vi "waypoint save to file.vi"() -> ()   [LabVIEW 2019]
panel:
  out "XY 그래프":cluster{"X":dbl, "Y":dbl}[](graph)
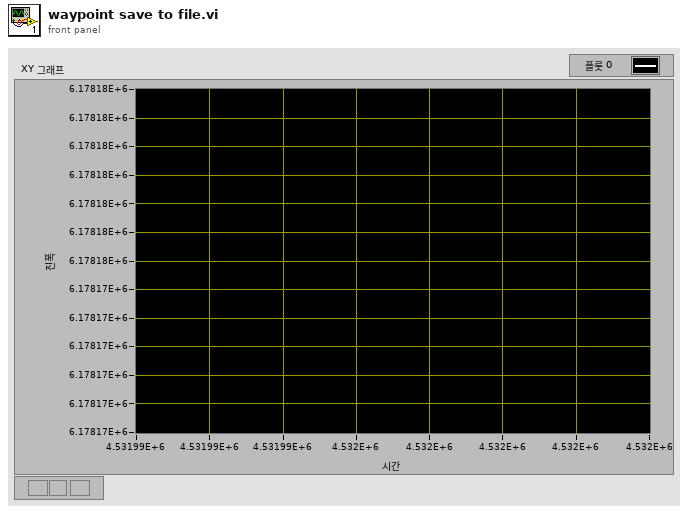
[diagram p1: front panel]
types:
  T1 = enum16{"open", "replace", "create", "open or create", "replace or create", "replace or create with confirmation"}
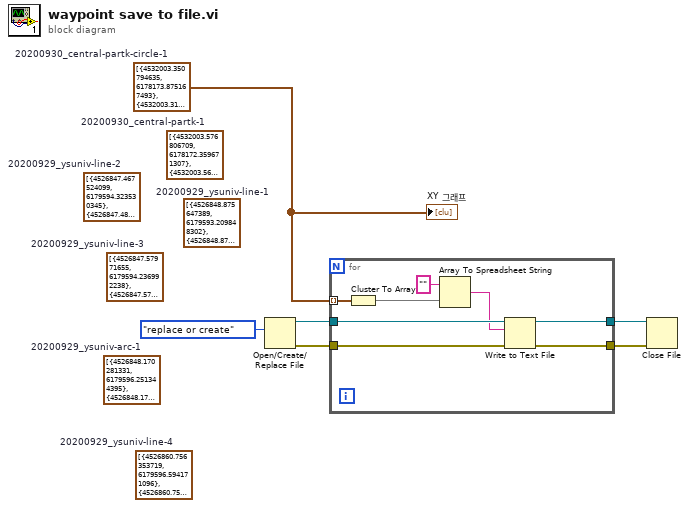
[diagram p0: block diagram]
diagram:
  w1 = cluster{"X":dbl, "Y":dbl}[] [{"X"=4532003.350794635, "Y"=6178173.875167493}, {"X"=4532003.318056276, "Y"=6178173.892770662}, {"X"=4532003.1579189105, "Y"=6178174.020957441}, {"X"=4532002.967709019, "Y"=6178174.196875582}, {"X"=4532002.672245268, "Y"=6178174.539853451}, {"X"=4532002.3370043775, "Y"=6178175.014684652}, {"X"=4532002.006206528, "Y"=6178175.539729376}, {"X"=4532001.675408691, "Y"=6178176.064773935}, {"X"=4532001.257877701, "Y"=6178176.578591164}, {"X"=4532000.912932229, "Y"=6178177.1375437835}, {"X"=4532000.552950506, "Y"=6178177.72036187}, {"X"=4532000.193857393, "Y"=6178178.313222488}, {"X"=4531999.835652887, "Y"=6178178.916125633}, {"X"=4531999.476559786, "Y"=6178179.508985873}, {"X"=4531998.959036802, "Y"=6178180.055525806}, {"X"=4531998.308713558, "Y"=6178180.457800657}, {"X"=4531997.609657364, "Y"=6178180.696909645}, {"X"=4531996.896383714, "Y"=6178180.775335258}, {"X"=4531996.09371134, "Y"=6178180.812405522}, {"X"=4531995.219342304, "Y"=6178180.814383002}, {"X"=4531994.477703708, "Y"=6178180.766033763}, {"X"=4531993.713031512, "Y"=6178180.651165896}, {"X"=4531992.935100371, "Y"=6178180.580249076}, {"X"=4531992.061620369, "Y"=6178180.592269521}, {"X"=4531991.173992895, "Y"=6178180.638198248}, {"X"=4531990.289920003, "Y"=6178180.724297736}, {"X"=4531989.372220418, "Y"=6178180.817957572}, {"X"=4531988.393487616, "Y"=6178180.997036841}, {"X"=4531987.627109124, "Y"=6178181.056675129}, {"X"=4531986.969538497, "Y"=6178180.989425519}, {"X"=4531986.427884561, "Y"=6178180.875629432}, {"X"=4531985.817199784, "Y"=6178180.75686876}, {"X"=4531985.116227672, "Y"=6178180.586710377}, {"X"=4531984.448882404, "Y"=6178180.408991751}, {"X"=4531983.6541389, "Y"=6178180.341855931}, {"X"=4531982.97797792, "Y"=6178180.258301622}, {"X"=4531982.517725303, "Y"=6178180.095477112}, {"X"=4531982.130876179, "Y"=6178179.793239902}, {"X"=4531982.0643702205, "Y"=6178179.429221983}, {"X"=4531982.268655881, "Y"=6178179.024806436}, {"X"=4531982.716326828, "Y"=6178178.6578521365}, {"X"=4531983.194958756, "Y"=6178178.253209357}, {"X"=4531983.691292785, "Y"=6178177.854828909}, {"X"=4531984.013272379, "Y"=6178177.4239516035}, {"X"=4531984.440575617, "Y"=6178177.020606336}, {"X"=4531984.7652211515, "Y"=6178176.619856802}, {"X"=4531985.021724419, "Y"=6178176.224185293}, {"X"=4531985.4543595435, "Y"=6178175.881095707}, {"X"=4531985.720637784, "Y"=6178175.595893426}, {"X"=4531986.162159305, "Y"=6178175.353230416}, {"X"=4531986.617828416, "Y"=6178175.076659101}, {"X"=4531987.01861415, "Y"=6178174.761214936}, {"X"=4531987.26185866, "Y"=6178174.409493832}, {"X"=4531987.470587696, "Y"=6178174.0552904}, {"X"=4531987.62887644, "Y"=6178173.71242755}, {"X"=4531987.941151956, "Y"=6178173.365670737}, {"X"=4531988.396821304, "Y"=6178173.089098919}, {"X"=4531989.048102098, "Y"=6178172.891456849}, {"X"=4531989.779077613, "Y"=6178172.8192914985}, {"X"=4531990.564048076, "Y"=6178172.775956259}, {"X"=4531991.397681722, "Y"=6178172.701194981}, {"X"=4531992.151691418, "Y"=6178172.6955483295}, {"X"=4531992.878294688, "Y"=6178172.767761083}, {"X"=4531993.734073901, "Y"=6178172.749475895}, {"X"=4531994.601334941, "Y"=6178172.667154285}, {"X"=4531995.4986685645, "Y"=6178172.537101383}, {"X"=4531996.445554117, "Y"=6178172.385665071}, {"X"=4531997.164160308, "Y"=6178172.367493635}, {"X"=4531997.672189098, "Y"=6178172.488849631}, {"X"=4531998.035117029, "Y"=6178172.714526736}, {"X"=4531998.284793752, "Y"=6178173.016879048}, {"X"=4531998.345079205, "Y"=6178173.310600223}, {"X"=4531998.336333534, "Y"=6178173.599356818}, {"X"=4531998.326628996, "Y"=6178173.683478796}, {"X"=4531998.2930020625, "Y"=6178173.691039228}, {"X"=4531998.374403547, "Y"=6178173.642009985}, {"X"=4531999.008942478, "Y"=6178173.642740035}, {"X"=4531999.9470125865, "Y"=6178173.585468922}, {"X"=4532000.815163115, "Y"=6178173.513190527}, {"X"=4532001.679759347, "Y"=6178173.400741216}, {"X"=4532002.4736174755, "Y"=6178173.457834008}, {"X"=4532003.167483395, "Y"=6178173.5476509305}, {"X"=4532003.230364361, "Y"=6178173.67690859}, {"X"=4532003.0135662975, "Y"=6178173.746136882}, {"X"=4532002.899426356, "Y"=6178173.812769338}, {"X"=4532002.781731981, "Y"=6178173.839230853}, {"X"=4532002.700330401, "Y"=6178173.888260139}, {"X"=4532002.602115337, "Y"=6178173.9410696365}, {"X"=4532002.537527241, "Y"=6178173.986318699}, {"X"=4532002.539304456, "Y"=6178174.006404166}, {"X"=4532002.557895154, "Y"=6178174.022709415}, {"X"=4532002.57648585, "Y"=6178174.039014672}, {"X"=4532002.594187939, "Y"=6178174.0452771885}]  # 20200930_central-partk-circle-1
  (unwired) cluster{"X":dbl, "Y":dbl}[] [{"X"=4532003.576806709, "Y"=6178172.359671307}, {"X"=4532003.561770444, "Y"=6178172.383537013}, {"X"=4532003.192762356, "Y"=6178172.4767447}, {"X"=4532002.509629774, "Y"=6178172.702033042}, {"X"=4532001.58140402, "Y"=6178173.064366489}, {"X"=4532000.6080697365, "Y"=6178173.498296774}, {"X"=4531999.621476697, "Y"=6178173.97617793}, {"X"=4531998.631329475, "Y"=6178174.413887931}, {"X"=4531997.607555584, "Y"=6178174.8591581}, {"X"=4531996.653701655, "Y"=6178175.319435316}, {"X"=4531995.644075927, "Y"=6178175.730796639}, {"X"=4531994.618525636, "Y"=6178176.15598064}, {"X"=4531993.592975622, "Y"=6178176.581164397}, {"X"=4531992.5329104, "Y"=6178177.003865606}, {"X"=4531991.489658902, "Y"=6178177.422786382}, {"X"=4531990.527809001, "Y"=6178177.792677899}, {"X"=4531990.226944478, "Y"=6178177.880806713}, {"X"=4531990.291532346, "Y"=6178177.835557892}, {"X"=4531990.903854542, "Y"=6178177.585221218}, {"X"=4531991.817041466, "Y"=6178177.246755574}, {"X"=4531992.795705138, "Y"=6178176.873083589}, {"X"=4531993.754001148, "Y"=6178176.463020804}, {"X"=4531994.714074643, "Y"=6178176.073043199}, {"X"=4531995.743179421, "Y"=6178175.688029997}, {"X"=4531996.772284476, "Y"=6178175.303016582}, {"X"=4531997.801389806, "Y"=6178174.918002955}, {"X"=4531998.829606799, "Y"=6178174.5229464}, {"X"=4531999.824197129, "Y"=6178174.135450053}, {"X"=4532000.801974246, "Y"=6178173.751733712}, {"X"=4532001.763826745, "Y"=6178173.381840121}, {"X"=4532002.707977389, "Y"=6178173.005683826}, {"X"=4532003.204384415, "Y"=6178172.801892536}, {"X"=4532003.252159043, "Y"=6178172.760423654}, {"X"=4532003.199941362, "Y"=6178172.751678849}, {"X"=4532003.165425786, "Y"=6178172.749196558}, {"X"=4532003.130910202, "Y"=6178172.746714265}]  # 20200930_central-partk-1
  (unwired) cluster{"X":dbl, "Y":dbl}[] [{"X"=4526860.756353719, "Y"=6179596.594171096}, {"X"=4526860.756353719, "Y"=6179596.594171096}, {"X"=4526860.789939688, "Y"=6179596.586628506}, {"X"=4526860.805839669, "Y"=6179596.572834014}, {"X"=4526860.720981763, "Y"=6179596.581667278}, {"X"=4526860.416922099, "Y"=6179596.629504165}, {"X"=4526859.860967764, "Y"=6179596.733910446}, {"X"=4526859.07080483, "Y"=6179596.901137997}, {"X"=4526858.199356166, "Y"=6179597.1172915315}, {"X"=4526857.262521803, "Y"=6179597.368576525}, {"X"=4526856.323008658, "Y"=6179597.589791859}, {"X"=4526855.407258622, "Y"=6179597.693209538}, {"X"=4526854.471143788, "Y"=6179597.760305785}, {"X"=4526853.586300991, "Y"=6179597.826111375}, {"X"=4526852.740402278, "Y"=6179597.944513448}, {"X"=4526851.791960003, "Y"=6179598.065496877}, {"X"=4526850.8381598815, "Y"=6179598.12634129}, {"X"=4526849.881680892, "Y"=6179598.157116253}, {"X"=4526848.997731885, "Y"=6179598.232945081}, {"X"=4526848.085555225, "Y"=6179598.376455428}, {"X"=4526847.088521079, "Y"=6179598.528798994}, {"X"=4526846.057008274, "Y"=6179598.678661943}, {"X"=4526845.107674283, "Y"=6179598.78962218}, {"X"=4526844.836308457, "Y"=6179598.819893221}, {"X"=4526844.836308457, "Y"=6179598.819893221}, {"X"=4526844.852208359, "Y"=6179598.8060988}]  # 20200929_ysuniv-line-4
  (unwired) cluster{"X":dbl, "Y":dbl}[] [{"X"=4526848.170281331, "Y"=6179596.251344395}, {"X"=4526848.172067365, "Y"=6179596.271390712}, {"X"=4526848.174746415, "Y"=6179596.301460189}, {"X"=4526848.193325387, "Y"=6179596.317735211}, {"X"=4526848.19511142, "Y"=6179596.337781527}, {"X"=4526848.318020094, "Y"=6179596.371521415}, {"X"=4526848.567409516, "Y"=6179596.479093841}, {"X"=4526849.057258204, "Y"=6179596.594007136}, {"X"=4526849.650543608, "Y"=6179596.716362219}, {"X"=4526850.3931795405, "Y"=6179596.784729416}, {"X"=4526851.303745028, "Y"=6179596.815383756}, {"X"=4526852.1675038235, "Y"=6179596.897444746}, {"X"=4526852.889949204, "Y"=6179597.1237023715}, {"X"=4526853.4180231765, "Y"=6179597.475401011}, {"X"=4526853.861239307, "Y"=6179597.835933031}, {"X"=4526854.190476694, "Y"=6179598.262956845}, {"X"=4526854.501135052, "Y"=6179598.673705659}, {"X"=4526854.860386211, "Y"=6179599.053094346}, {"X"=4526855.3195020575, "Y"=6179599.399832276}, {"X"=4526855.828103734, "Y"=6179599.725233304}, {"X"=4526856.067125019, "Y"=6179600.100951621}, {"X"=4526856.206281487, "Y"=6179600.509320781}, {"X"=4526856.273801102, "Y"=6179600.882659113}, {"X"=4526856.14945422, "Y"=6179601.217295914}, {"X"=4526855.675134219, "Y"=6179601.661198722}, {"X"=4526855.062005723, "Y"=6179602.085155568}, {"X"=4526854.368310677, "Y"=6179602.373849684}, {"X"=4526853.501328359, "Y"=6179602.640117238}, {"X"=4526852.607730369, "Y"=6179602.799901114}, {"X"=4526851.800602298, "Y"=6179602.776686818}, {"X"=4526851.081730017, "Y"=6179602.590520808}, {"X"=4526850.492736272, "Y"=6179602.324069063}, {"X"=4526850.067206864, "Y"=6179601.9697890505}, {"X"=4526849.843192611, "Y"=6179601.570253982}, {"X"=4526849.956823016, "Y"=6179601.115339965}, {"X"=4526849.968802758, "Y"=6179600.673030329}, {"X"=4526849.760688252, "Y"=6179600.259700865}, {"X"=4526849.320151586, "Y"=6179599.929238734}, {"X"=4526848.731157484, "Y"=6179599.662787635}, {"X"=4526848.168779378, "Y"=6179599.502820084}, {"X"=4526847.817739581, "Y"=6179599.407851984}, {"X"=4526847.179433946, "Y"=6179599.356949316}, {"X"=4526846.581684026, "Y"=6179599.184478212}, {"X"=4526846.227790916, "Y"=6179598.865229688}, {"X"=4526846.242449157, "Y"=6179598.452989891}, {"X"=4526846.59921707, "Y"=6179598.035486411}, {"X"=4526847.123021329, "Y"=6179597.570246789}, {"X"=4526847.458531307, "Y"=6179597.106398559}, {"X"=4526847.916056945, "Y"=6179596.666266938}, {"X"=4526848.549549199, "Y"=6179596.27863064}, {"X"=4526849.392594041, "Y"=6179595.935947071}, {"X"=4526850.155420726, "Y"=6179595.846423975}, {"X"=4526850.457693785, "Y"=6179595.778540601}, {"X"=4526850.523079555, "Y"=6179595.743409067}, {"X"=4526850.637058142, "Y"=6179595.676917302}, {"X"=4526850.734243783, "Y"=6179595.614196826}, {"X"=4526850.832322437, "Y"=6179595.561499524}, {"X"=4526850.895922179, "Y"=6179595.506321643}]  # 20200929_ysuniv-arc-1
  (unwired) cluster{"X":dbl, "Y":dbl}[] [{"X"=4526847.57971655, "Y"=6179594.236992238}, {"X"=4526847.578823527, "Y"=6179594.226969077}, {"X"=4526847.5779305035, "Y"=6179594.216945917}, {"X"=4526847.577037481, "Y"=6179594.206922759}, {"X"=4526847.817496807, "Y"=6179594.214263396}, {"X"=4526848.30377362, "Y"=6179594.28908366}, {"X"=4526848.877587275, "Y"=6179594.385140075}, {"X"=4526849.469979942, "Y"=6179594.49747158}, {"X"=4526850.149909467, "Y"=6179594.6310392935}, {"X"=4526850.917375851, "Y"=6179594.785843256}, {"X"=4526851.720214229, "Y"=6179594.953151071}, {"X"=4526852.541631642, "Y"=6179595.136734074}, {"X"=4526853.345363136, "Y"=6179595.314065338}, {"X"=4526854.151773704, "Y"=6179595.5214662915}, {"X"=4526854.942284363, "Y"=6179595.7426618785}, {"X"=4526855.729223025, "Y"=6179595.923764881}, {"X"=4526856.532061694, "Y"=6179596.091073533}, {"X"=4526857.301314478, "Y"=6179596.265924913}, {"X"=4526858.087360279, "Y"=6179596.437005135}, {"X"=4526858.874299126, "Y"=6179596.61810868}, {"X"=4526859.578166127, "Y"=6179596.828092018}, {"X"=4526860.330626089, "Y"=6179597.006715212}, {"X"=4526861.154722999, "Y"=6179597.22036939}, {"X"=4526861.497007489, "Y"=6179597.409318161}, {"X"=4526861.4528794885, "Y"=6179597.490794452}, {"X"=4526861.303528628, "Y"=6179597.544782445}, {"X"=4526861.2054497115, "Y"=6179597.597479778}, {"X"=4526861.072891846, "Y"=6179597.647696484}]  # 20200929_ysuniv-line-3
  (unwired) cluster{"X":dbl, "Y":dbl}[] [{"X"=4526847.467524099, "Y"=6179594.323530345}, {"X"=4526847.485210063, "Y"=6179594.329782201}, {"X"=4526847.502896027, "Y"=6179594.336034054}, {"X"=4526847.571853841, "Y"=6179594.340995139}, {"X"=4526847.697441634, "Y"=6179594.40480442}, {"X"=4526847.892880264, "Y"=6179594.483597957}, {"X"=4526848.236776315, "Y"=6179594.498380264}, {"X"=4526848.501172765, "Y"=6179594.582134931}, {"X"=4526848.667490617, "Y"=6179594.718586936}, {"X"=4526848.802901622, "Y"=6179594.892651054}, {"X"=4526848.939205637, "Y"=6179595.0767383445}, {"X"=4526849.057823673, "Y"=6179595.254573792}, {"X"=4526849.177334716, "Y"=6179595.442432413}, {"X"=4526849.329538613, "Y"=6179595.612725276}, {"X"=4526849.498535446, "Y"=6179595.779246859}, {"X"=4526849.732025003, "Y"=6179595.900613774}, {"X"=4526849.999100443, "Y"=6179596.014438112}, {"X"=4526850.33066864, "Y"=6179596.083107786}, {"X"=4526850.781573511, "Y"=6179596.145424739}, {"X"=4526851.3350221235, "Y"=6179596.2051602965}, {"X"=4526851.972435541, "Y"=6179596.246039417}, {"X"=4526852.642541916, "Y"=6179596.269352819}, {"X"=4526853.4125131, "Y"=6179596.260015311}, {"X"=4526854.168370443, "Y"=6179596.284518674}, {"X"=4526854.859735047, "Y"=6179596.354176823}, {"X"=4526855.454806941, "Y"=6179596.496578729}, {"X"=4526855.918214148, "Y"=6179596.699220611}, {"X"=4526856.253528623, "Y"=6179597.002195207}, {"X"=4526856.42269941, "Y"=6179597.36292913}, {"X"=4526856.44341244, "Y"=6179597.787674212}, {"X"=4526856.4171445295, "Y"=6179598.069614061}, {"X"=4526856.4412554875, "Y"=6179598.340240047}, {"X"=4526856.641333033, "Y"=6179598.66336188}, {"X"=4526857.121532972, "Y"=6179598.862232873}, {"X"=4526857.633532847, "Y"=6179599.0335150175}, {"X"=4526857.742327595, "Y"=6179599.101096036}, {"X"=4526857.677834711, "Y"=6179599.146250714}, {"X"=4526857.629241795, "Y"=6179599.177610924}, {"X"=4526857.581541879, "Y"=6179599.218994313}, {"X"=4526857.549741936, "Y"=6179599.246583243}, {"X"=4526857.500256033, "Y"=6179599.267920262}]  # 20200929_ysuniv-line-2
  (unwired) cluster{"X":dbl, "Y":dbl}[] [{"X"=4526848.875647389, "Y"=6179593.209848302}, {"X"=4526848.878326462, "Y"=6179593.239917798}, {"X"=4526848.898691504, "Y"=6179593.276239142}, {"X"=4526849.058758274, "Y"=6179593.342528971}, {"X"=4526849.445170584, "Y"=6179593.450000222}, {"X"=4526849.882854773, "Y"=6179593.556180745}, {"X"=4526850.441661731, "Y"=6179593.676054804}, {"X"=4526851.08443348, "Y"=6179593.777072374}, {"X"=4526851.7943771025, "Y"=6179593.863004775}, {"X"=4526852.537906699, "Y"=6179593.941394629}, {"X"=4526853.28232938, "Y"=6179594.02980775}, {"X"=4526854.001203319, "Y"=6179594.215972202}, {"X"=4526854.606098577, "Y"=6179594.468628661}, {"X"=4526855.01305027, "Y"=6179594.806633645}, {"X"=4526855.533980649, "Y"=6179595.07814685}, {"X"=4526856.187468742, "Y"=6179595.299443374}, {"X"=4526856.939928663, "Y"=6179595.478065833}, {"X"=4526857.7391955275, "Y"=6179595.605281743}, {"X"=4526857.952320257, "Y"=6179595.690327663}, {"X"=4526858.317474763, "Y"=6179595.7514550835}, {"X"=4526858.855917065, "Y"=6179595.835008726}, {"X"=4526859.448310326, "Y"=6179595.947341314}, {"X"=4526859.94173174, "Y"=6179596.102348155}, {"X"=4526860.47231111, "Y"=6179596.2899052715}, {"X"=4526861.089534393, "Y"=6179596.488675603}, {"X"=4526861.743915627, "Y"=6179596.719996271}, {"X"=4526862.364710898, "Y"=6179596.958859657}, {"X"=4526862.492977711, "Y"=6179597.052739102}, {"X"=4526862.461177725, "Y"=6179597.080328097}, {"X"=4526862.410798762, "Y"=6179597.091641968}, {"X"=4526862.343626815, "Y"=6179597.106727131}]  # 20200929_ysuniv-line-1
  n1 = Open/Create/Replace File(operation (0:open)=T1."replace or create" ("동작(0:open)")) -> (refnum out=w4:refnum<file>, error out=w6:errorcluster)  [unwired: 5 in, 1 out]
  n2 = for {
    tunnel: w6 -> [w14]
    tunnel: [w13] -> w5
    tunnel: w4 -> [w12]
    tunnel: [w11] -> w3
    tunnel: w1 -> [w10] mode=indexing
    n3 = Cluster To Array(cluster=w10) -> (array=w9:dbl[])
    n4 = Array To Spreadsheet String(array=w9, 3:"" ("포맷 문자열")) -> (spreadsheet string=w7:string)  [unwired: 1 in]
    n5 = Write to Text File(file (use dialog)=w12, text=w7, error in=w14) -> (refnum out=w11:refnum<file>, error out=w13:errorcluster)  [unwired: 1 in, 1 out]
  }
  n6 = Close File(refnum=w3, error in=w5) -> ()  [unwired: 2 out]
  "XY 그래프" <- w1
